vi "Test Auto_Navigate_1.vi"() -> ()   [LabVIEW 2011]
uses:
  Kinect_Raw_Depth_to_Meters_Double.vi
  Convert_Meters_to_Inches_Double.vi
panel:
  in  "horizontal_fov":sgl=60.0
  out "min_distance_index":i32=143
  in  "stop":bool
  in  "threshold":sgl=1000.0
  in  "strip_offset":sgl=147.0
  in  "strip_width":sgl=5.0
  out "steering_angle":sgl
  out "minimum_distance":sgl=275.03433
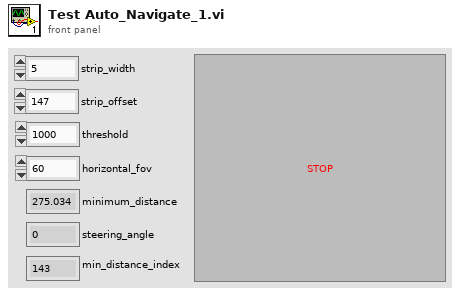
[diagram p1: front panel]
types:
  T1 = typedef "Image Type" = u32
  T2 = typedef "IMAQ Image.ctl" = refnum<image>
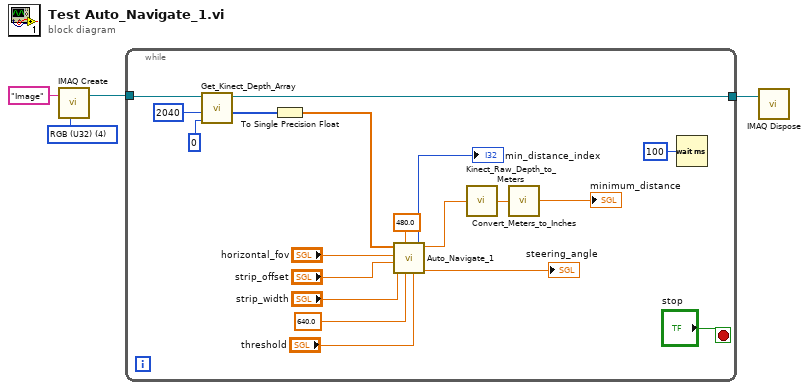
[diagram p0: block diagram]
diagram:
  w1 = T1 4 items=["Grayscale (U8)", "Grayscale (I16)", "Grayscale (SGL)", "Complex (CSG)", "RGB (U32)", "HSL (U32)", "RGB (U64)", "Grayscale (U16)"] ("Image Type")
  n1 = call "IMAQ Create"("Image Name"="Image", "Image Type"=w1) -> ("New Image"=w3:T2)  [unwired: 3 in, 1 out]
  n2 = while {
    tunnel: [w15] -> w4
    tunnel: w3 -> [w12]
    stop <- "stop" stop-if-true
    n3 = call "Get_Kinect_Depth_Array.vi"("Index"=0, "Far_Clip_Plane"=u16 2040, "Refnum_in"=w12) -> ("1D_Array"=w11:u16[], "Refnum_out"=w15:T2)  [unwired: 5 in, 2 out]
    n4 = To Single Precision Float(number=w11) -> (single precision float=w10:sgl[])
    n5 = call "Auto_Navigate_1.vi"("far_clip_value"="threshold", "columns"=sgl 640.0, "rows"=sgl 480.0, "strip_width"="strip_width", "strip_offset"="strip_offset", "horizontal_fov"="horizontal_fov", "distance_array"=w10) -> ("steering_angle"=→"steering_angle":sgl, "min_distance"=w9:sgl, "min_distance_index"=→"min_distance_index":i32)  [unwired: 2 in]
    n6 = call-poly "Kinect_Raw_Depth_to_Meters.vi"("Raw"=w9) -> ("Meters"=w8:dbl)  [unwired: 4 in]
    n7 = call-poly "Convert_Meters_to_Inches.vi"("Meters"=w8) -> ("Inches"=→"minimum_distance":dbl)  [unwired: 4 in]
    n8 = Wait (ms)(milliseconds to wait=u32 100) -> ()  [unwired: 1 out]
  }
  n9 = call "IMAQ Dispose"("Image"=w4) -> ()  [unwired: 5 in, 1 out]
